vi "Edit IDM Desc Array.vi"(11 "IDM Descriptor Array In":T1) -> (3 "IDM Descriptor Array Out":T1)   [LabVIEW 2021]
uses:
  <vilib>/myRIO/Common/Express VI Framework/typedefs/Instrument Driver Method Descriptor Array.ctl
  <vilib>/myRIO/Common/Express VI Framework/typedefs/Instrument Driver Method Descriptor.ctl
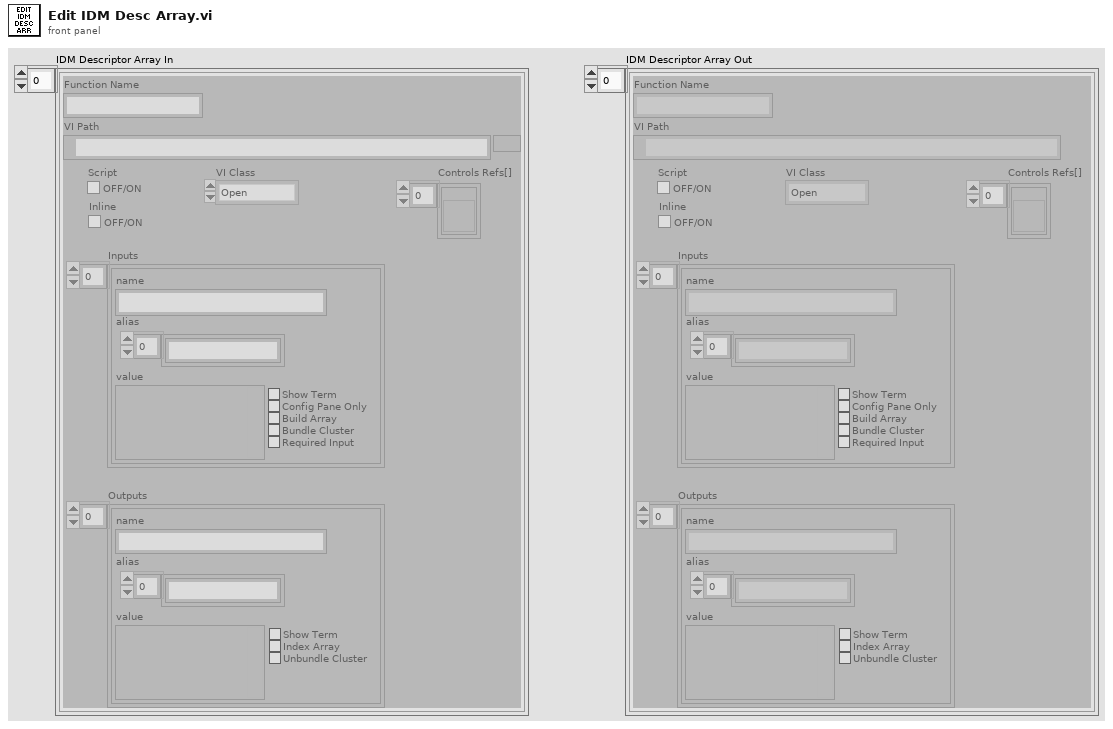
[diagram p1: front panel]
types:
  T1 = typedef "Instrument Driver Method Descriptor Array.ctl" = T2[]
  T2 = typedef "Instrument Driver Method Descriptor.ctl" = cluster{"Function Name":string, "VI Path":path, "Script":bool, "Inputs":cluster{"name":string, "value":variant, "Config Pane Only":bool, "Build Array":bool, "Bundle Cluster":bool, "Show Term":bool, "alias":string[], "Required Input":bool}[], "Outputs":cluster{"name":string, "value":variant, "Show Term":bool, "Index Array":bool, "Unbundle Cluster":bool, "alias":string[]}[], "VI Class":enum16{"Open", "Configure", "Data", "Manage", "Close"}, "Controls Refs[]":refnum<vi>[], "Inline":bool}
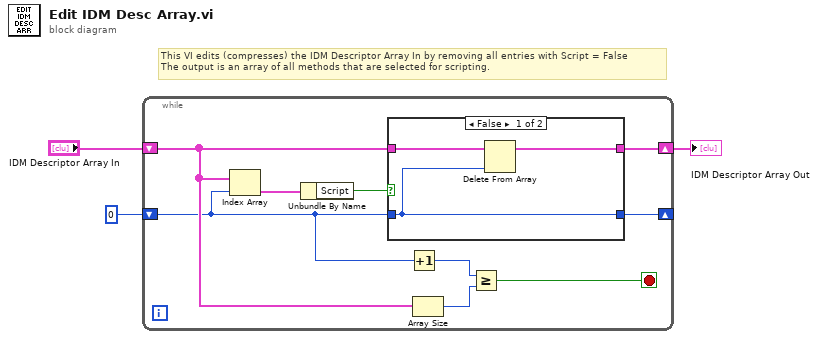
[diagram p0: block diagram]
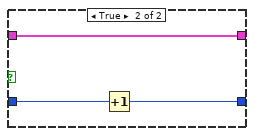
[diagram p2: hidden frame]
diagram:
  # "This VI edits (compresses) the IDM Descriptor Array In by removing all entries with Script = False\nThe output is an array of all methods that are selected for scripting."
  n1 = while {
    shift-right: [w12] -> _
    shift-left: 0 ("index") -> [w9]
    shift-right: [w11] -> w2
    shift-left: "IDM Descriptor Array In" -> [w10]
    stop <- w6 stop-if-true
    n2 = Index Array(array=w10, index=w9) -> (element=w5:T2)
    n3 = Unbundle By Name(w5) -> ("Script"=w4:bool)
    n4 = case shown="False" w4 {
      tunnel: w9 -> [w13 w18]
      tunnel: [w13 w17] -> w12
      tunnel: w10 -> [w15 w16]
      tunnel: [w14 w16] -> w11
      frame False {
        n5 = Delete From Array(array=w15, index=w13) -> (array with subset deleted=w14:T1)  [unwired: 1 in, 1 out]
      }
      frame True {
        n6 = Increment(x=w18) -> (x+1=w17:i32)
      }
    }
    n7 = Increment(x=w9) -> (x+1=w8:i32)
    n8 = Array Size(array=w10) -> (size(s)=w7:i32)
    n9 = Greater Or Equal?(x=w8, y=w7) -> (x >= y?=w6:bool)
  }
  "IDM Descriptor Array Out" <- w2
